vi "niFpgaPID_PIDStatelessCore.vi"(0 "errors":T2 {"error" step=0.125}, 1 "reset? (F)":bool, 5 "enable bumpless transfer? (F)":bool, 7 "manual control":T6, 11 "state in":T3, 12 "gains":T4 {"filter coefficient" min=0 max=1; "proportional gain" step=0.125}, 13 "output range":T5={"output high (Inf)"=inf, "output low (-Inf)"=-inf}) -> (4 "output":sgl, 6 "error":sgl, 8 "actions":T1, 15 "state out":T3)   [LabVIEW 2017]
uses:
  <vilib>/rvi/Analysis/control/PID/Typedef/niFpgaPID_ManualControl.ctl
  <vilib>/rvi/Analysis/control/PID/Typedef/niFpgaPID_OutputRange.ctl
  <vilib>/rvi/Analysis/control/PID/Typedef/niFpgaPID_PIDGains.ctl
  <vilib>/rvi/Analysis/control/PID/Typedef/niFpgaPID_PIDState.ctl
  <vilib>/rvi/Analysis/control/PID/Typedef/niFpgaPID_PIDErrors.ctl
  <vilib>/rvi/Analysis/control/PID/Typedef/niFpgaPID_PIDActions.ctl
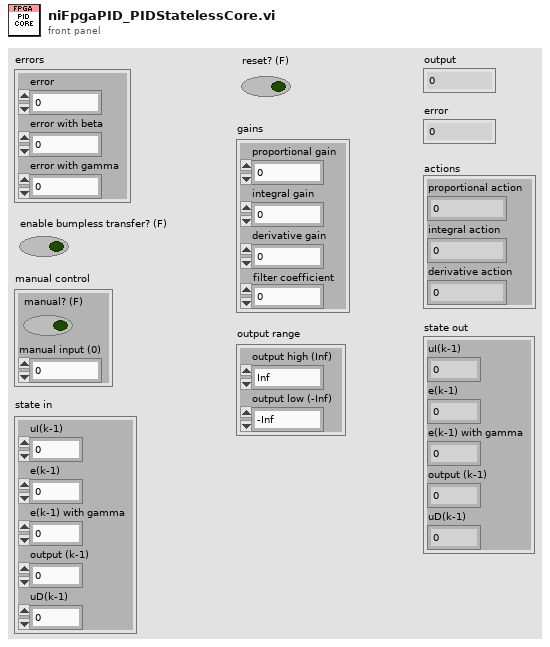
[diagram p1: front panel]
types:
  T1 = typedef "niFpgaPID_PIDActions.ctl" = cluster{"proportional action":sgl, "integral action":sgl, "derivative action":sgl}
  T2 = typedef "niFpgaPID_PIDErrors.ctl" = cluster{"error":sgl, "error with beta":sgl, "error with gamma":sgl}
  T3 = typedef "niFpgaPID_PIDState.ctl" = cluster{"uI(k-1)":sgl, "e(k-1)":sgl, "e(k-1) with gamma":sgl, "output (k-1)":sgl, "uD(k-1)":sgl}
  T4 = typedef "niFpgaPID_PIDGains.ctl" = cluster{"proportional gain":sgl, "integral gain":sgl, "derivative gain":sgl, "filter coefficient":sgl}
  T5 = typedef "niFpgaPID_OutputRange.ctl" = cluster{"output high (Inf)":sgl, "output low (-Inf)":sgl}
  T6 = typedef "niFpgaPID_ManualControl.ctl" = cluster{"manual? (F)":bool, "manual input (0)":sgl}
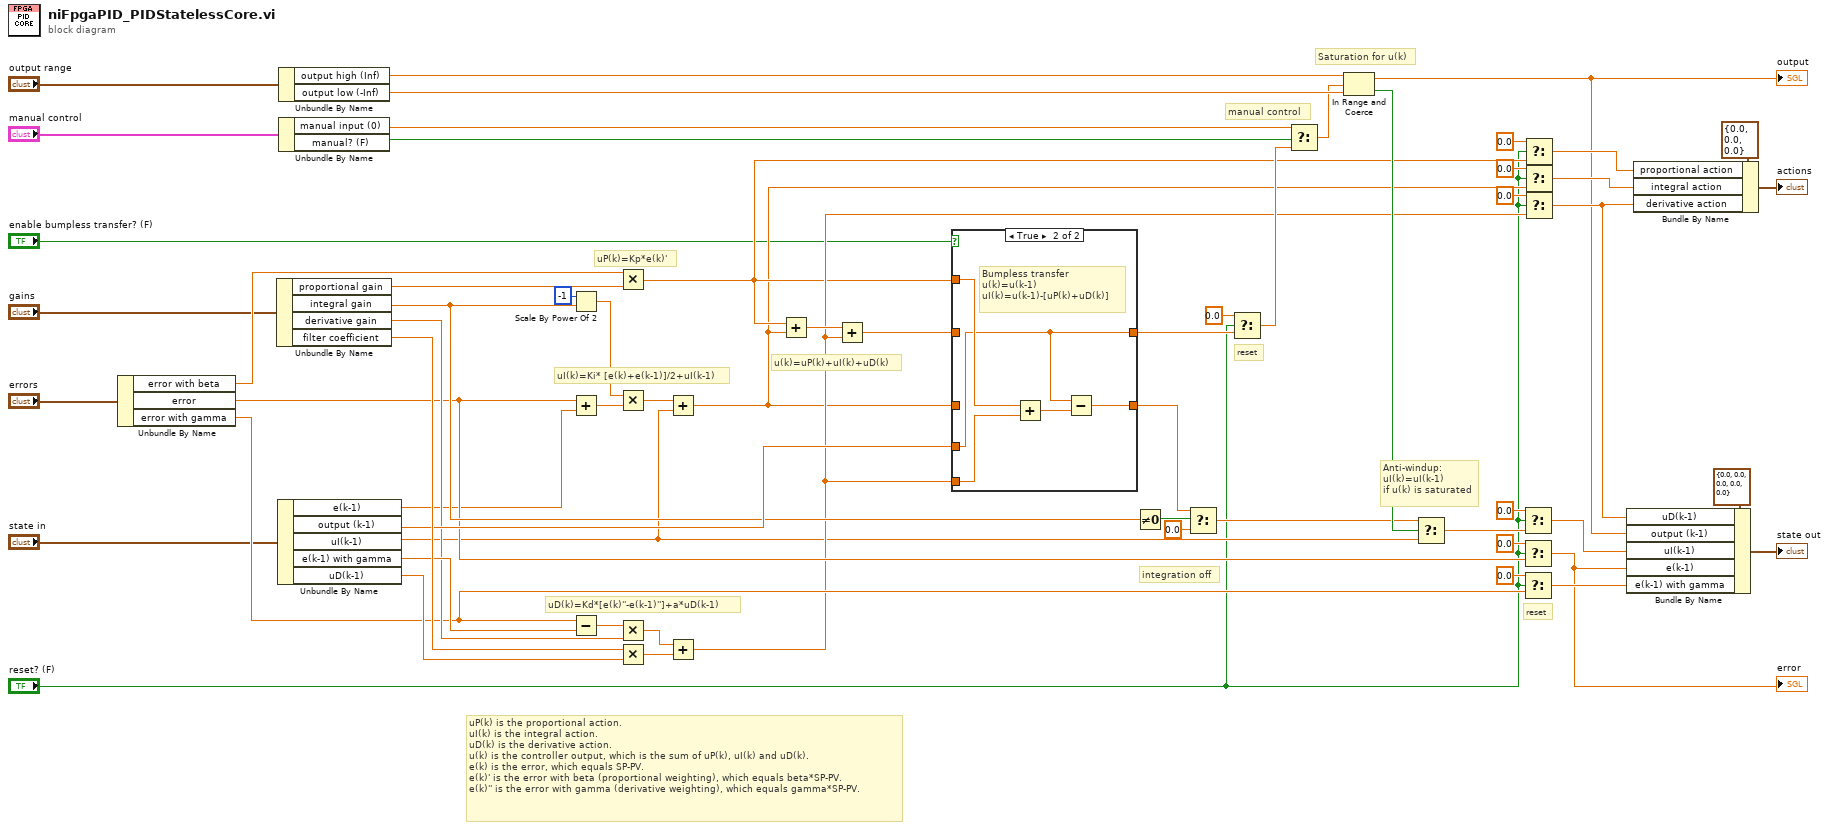
[diagram p0: block diagram]
diagram:
  # "uP(k) is the proportional action.\nuI(k) is the integral action.\nuD(k) is the derivative action.\nu(k) is the controller output, which is the sum of uP(k), uI(k) and uD(k).\ne(k) is the error, which equals SP-PV.\ne(k)' is the error with beta (proportional weighting), which equals beta*SP-PV.\ne(k)'' is the error with gamma (derivative weighting), which equals gamma*SP-PV."
  # "manual control"
  # "reset"
  # "reset"
  # "integration off"
  # "u(k)=uP(k)+uI(k)+uD(k)"
  # "uI(k)=Ki* [e(k)+e(k-1)]/2+uI(k-1)"
  # "uD(k)=Kd*[e(k)''-e(k-1)'']+a*uD(k-1)"
  # "uP(k)=Kp*e(k)'"
  # "Anti-windup:\nuI(k)=uI(k-1) \nif u(k) is saturated"
  # "Saturation for u(k)"
  n1 = Unbundle By Name("errors") -> ("error with beta"=w49:sgl, "error"=w27:sgl, "error with gamma"=w25:sgl)
  n2 = Unbundle By Name("gains") -> ("proportional gain"=w51:sgl, "integral gain"=w40:sgl, "derivative gain"=w42:sgl, "filter coefficient"=w56:sgl)
  n3 = Unbundle By Name("state in") -> ("e(k-1)"=w13:sgl, "output (k-1)"=w50:sgl, "uI(k-1)"=w12:sgl, "e(k-1) with gamma"=w48:sgl, "uD(k-1)"=w55:sgl)
  n4 = Unbundle By Name("output range") -> ("output high (Inf)"=w61:sgl, "output low (-Inf)"=w60:sgl)
  n5 = Unbundle By Name("manual control") -> ("manual input (0)"=w39:sgl, "manual? (F)"=w38:bool)
  n6 = Scale By Power Of 2(n=i16 -1, x=w40) -> (x*2^n=w45:sgl)
  n7 = Add(x=w27, y=w13) -> (x+y=w46:sgl)
  n8 = Subtract(x=w25, y=w48) -> (x-y=w54:sgl)
  n9 = Multiply(x=w49, y=w51) -> (x*y=w16:sgl)
  n10 = Multiply(x=w45, y=w46) -> (x*y=w58:sgl)
  n11 = Multiply(x=w54, y=w42) -> (x*y=w53:sgl)
  n12 = Multiply(x=w56, y=w55) -> (x*y=w52:sgl)
  n13 = Add(x=w58, y=w12) -> (x+y=w15:sgl)
  n14 = Add(x=w53, y=w52) -> (x+y=w21:sgl)
  n15 = Add(x=w16, y=w15) -> (x+y=w57:sgl)
  n16 = Add(x=w57, y=w21) -> (x+y=w37:sgl)
  n17 = case shown="True" "enable bumpless transfer? (F)" {
    tunnel: w37 -> [w64 _]
    tunnel: [w64 w65] -> w33
    tunnel: w15 -> [w63 _]
    tunnel: [w63 w69] -> w44
    tunnel: w16 -> [_ w68]
    tunnel: w50 -> [_ w65]
    tunnel: w21 -> [_ w66]
    frame False {
    }
    frame True {
      # "Bumpless transfer\nu(k)=u(k-1)\nuI(k)=u(k-1)-[uP(k)+uD(k)]"
      n18 = Add(x=w68, y=w66) -> (x+y=w67:sgl)
      n19 = Subtract(x=w65, y=w67) -> (x-y=w69:sgl)
    }
  }
  n20 = Not Equal To 0?(x=w40) -> (x != 0?=w41:bool)
  n21 = Select(t=w44, s=w41, f=sgl 0.0) -> (s? t:f=w35:sgl)
  n22 = Select(t=sgl 0.0, s="reset? (F)", f=w33) -> (s? t:f=w34:sgl)
  n23 = Select(t=w39, s=w38, f=w34) -> (s? t:f=w59:sgl)
  n24 = In Range and Coerce(upper limit=w61, x=w59, lower limit=w60) -> (coerced(x)=w4:sgl, In Range?=w62:bool)
  "output" <- w4
  n25 = Select(t=w35, s=w62, f=w12) -> (s? t:f=w29:sgl)
  n26 = Select(t=sgl 0.0, s="reset? (F)", f=w29) -> (s? t:f=w30:sgl)
  n27 = Select(t=sgl 0.0, s="reset? (F)", f=w27) -> (s? t:f=w1:sgl)
  "error" <- w1
  n28 = Select(t=sgl 0.0, s="reset? (F)", f=w25) -> (s? t:f=w24:sgl)
  n29 = Select(t=sgl 0.0, s="reset? (F)", f=w16) -> (s? t:f=w17:sgl)
  n30 = Select(t=sgl 0.0, s="reset? (F)", f=w15) -> (s? t:f=w14:sgl)
  n31 = Select(t=sgl 0.0, s="reset? (F)", f=w21) -> (s? t:f=w20:sgl)
  n32 = Bundle By Name(cluster=T3 {"uI(k-1)"=0.0, "e(k-1)"=0.0, "e(k-1) with gamma"=0.0, "output (k-1)"=0.0, "uD(k-1)"=0.0} ("state"), "uD(k-1)"=w20, "output (k-1)"=w4, "uI(k-1)"=w30, "e(k-1)"=w1, "e(k-1) with gamma"=w24) -> (→"state out":T3)
  n33 = Bundle By Name(cluster=T1 {"proportional action"=0.0, "integral action"=0.0, "derivative action"=0.0} ("actions"), "proportional action"=w17, "integral action"=w14, "derivative action"=w20) -> (→"actions":T1)
